vi "update values.vi"(11 "register values":u16[](array[numeric])) -> (3 "register":u16)   [LabVIEW 2021]
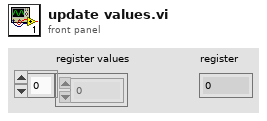
[diagram p1: front panel]
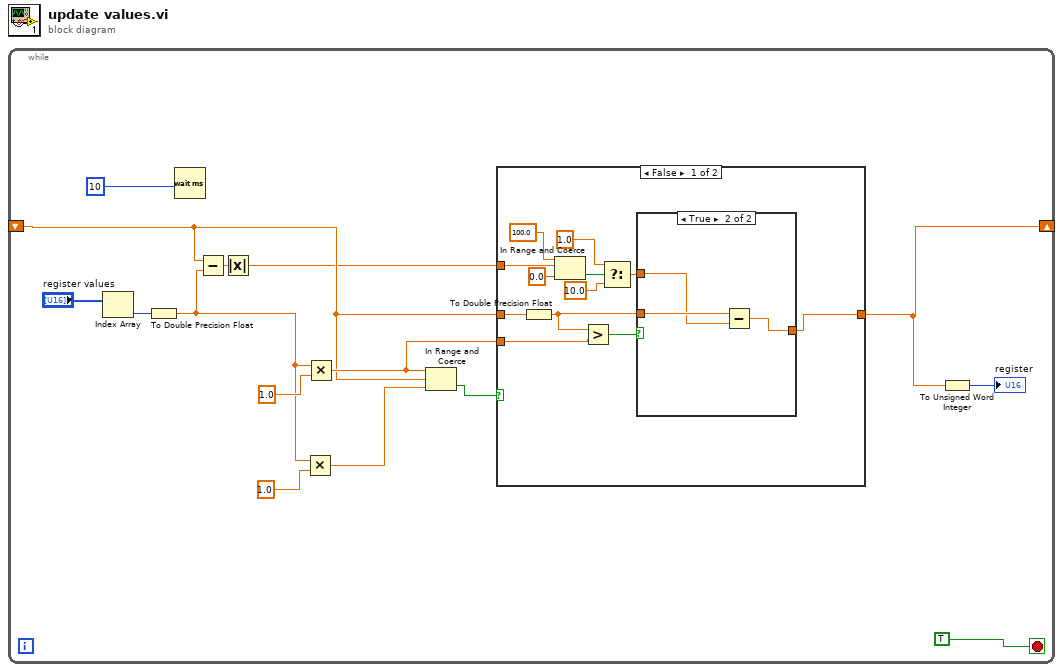
[diagram p0: block diagram]
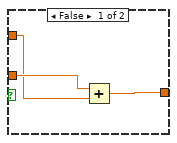
[diagram p2: hidden frame]
diagram:
  n1 = while {
    shift-right: [w6] -> _
    shift-left: _ -> [w9]
    stop <- TRUE ("Boolean") stop-if-true
    n2 = Index Array(array="register values") -> (element=w8:u16)  [unwired: 1 in]
    n3 = To Double Precision Float(number=w8) -> (double precision float=w5:dbl)
    n4 = Wait (ms)(milliseconds to wait=u32 10) -> ()  [unwired: 1 out]
    n5 = Subtract(x=w9, y=w5) -> (x-y=w4:dbl)
    n6 = Absolute Value(x=w4) -> (abs(x)=w1:dbl)
    n7 = Multiply(x=w5, y=1.0) -> (x*y=w12:dbl)
    n8 = Multiply(x=w5, y=1.0) -> (x*y=w10:dbl)
    n9 = In Range and Coerce(upper limit=w10, x=w9, lower limit=w12) -> (In Range?=w11:bool)  [unwired: 1 out]
    n10 = case shown="False" w11 {
      tunnel: [w23 w34] -> w6
      tunnel: w10 -> [w27 _]
      tunnel: w9 -> [w24 w34]
      tunnel: w1 -> [w22 _]
      frame False {
        n11 = To Double Precision Float(number=w24) -> (double precision float=w25:dbl)
        n12 = In Range and Coerce(upper limit=100.0, x=w22, lower limit=0.0) -> (In Range?=w19:bool)  [unwired: 1 out]
        n13 = Greater?(x=w25, y=w27) -> (0:w26:bool)
        n14 = Select(t=1.0, s=w19, f=10.0) -> (s? t:f=w17:dbl)
        n15 = case shown="True" w26 {
          tunnel: w25 -> [w29 w32]
          tunnel: [w30 w33] -> w23
          tunnel: w17 -> [w28 w31]
          frame False {
            n16 = Add(x=w29, y=w28) -> (x+y=w30:dbl)
          }
          frame True {
            n17 = Subtract(x=w32, y=w31) -> (x-y=w33:dbl)
          }
        }
      }
      frame True {
      }
    }
    n18 = To Unsigned Word Integer(number=w6) -> (unsigned 16bit integer=→"register":u16)
  }
